vi "StockFPGA_InlinedNotRioSessionBit.vi"() -> (0 "Not RIO Session Bit":u32=8192)   [LabVIEW 2017]
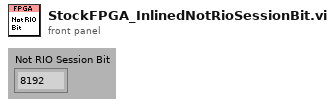
[diagram p1: front panel]
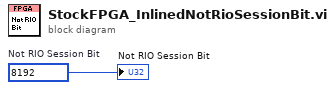
[diagram p0: block diagram]
diagram:
  w1 = u32 8192  # Not RIO Session Bit
  "Not RIO Session Bit" <- w1
